vi "IMAQ FPGA Camera Link Falling Edge Detect.vi"(10 "Input Valid":bool=TRUE, 11 "Input":bool) -> (3 "Falling Edge":bool)   [LabVIEW 2017]
doc: "This VI generates a single-cycle pulse each time there is a high-to-low transition on the input signal. This makes it easy to detect falling edges on signals."
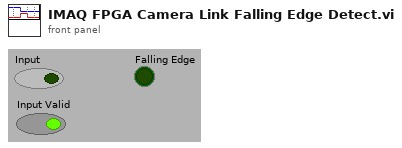
[diagram p1: front panel]
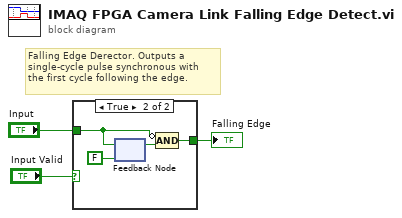
[diagram p0: block diagram]
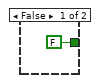
[diagram p2: hidden frame]
diagram:
  # "Falling Edge Derector. Outputs a\nsingle-cycle pulse synchronous with\nthe first cycle following the edge."
  n1 = case shown="True" "Input Valid" {
    tunnel: "Input" -> [_ w6]
    tunnel: [FALSE w5] -> w2
    frame False {
    }
    frame True {
      n2 = feedback #1(FALSE ("FV")) -> (w7:bool)
      n3 = feedback-in #1(w6) -> ()
      n4 = Compound Arithmetic op=AND(invert w6, w7) -> (w5:bool)
    }
  }
  "Falling Edge" <- w2
